vi "基于LabVIEW的光照度监测系统上位机软件设计.vi"() -> ()   [LabVIEW 2025]
uses:
  <vilib>/Instr/_visa.llb/VISA Configure Serial Port (Instr).vi
panel:
  out "转换为十进制数据":u32
  out "地址04的光亮度数据":dbl
  out "字符串显示·的十六进制数据":string
  out "无符号字节数组":u8[](array[numeric])
  out "十六进制整形字符串":string[](array[string])
  out "提取的从机地址04的亮度原始数据":string
  out "转换为十进制数据":u32
  out "地址03的光亮度数据":dbl
  out "字符串显示·的十六进制数据":string
  out "无符号字节数组":u8[](array[numeric])
  out "十六进制整形字符串":string[](array[string])
  out "提取的从机地址03的亮度原始数据":string
  out "转换为十进制数据":u32
  out "地址02的光亮度数据":dbl
  out "字符串显示的十六进制数据":string
  out "无符号字节数组":u8[](array[numeric])
  out "十六进制整形字符串":string[](array[string])
  out "提取的从机地址02的亮度原始数据":string
  out "转换为十进制数据":u32
  out "地址01的光亮度数据":dbl
  out "字符串显示的十六进制数据":string
  out "无符号字节数组":u8[](array[numeric])
  out "十六进制整形字符串":string[](array[string])
  out "提取的从机地址01的亮度原始数据":string
  out "地址03":u32(graph)
  out "地址04":u32(graph)
  in  "选择从机":u16(ring)=4 items=["从机04"=4, "从机03"=3, "从机02"=2, "从机01"=1]
  out "地址02":u32(graph)
  out "地址01":u32(graph)
  in  "停止采集":bool
  out "所有测量记录":string[][](table)
  in  "发送命令":string
  in  "波特率":u32=9600 caption="波特率(9600)"
  in  "选择串口":refnum<visa-resource-name>
  # "从机地址01："
  # "从机地址02："
  # "从机地址03："
  # "从机地址04："
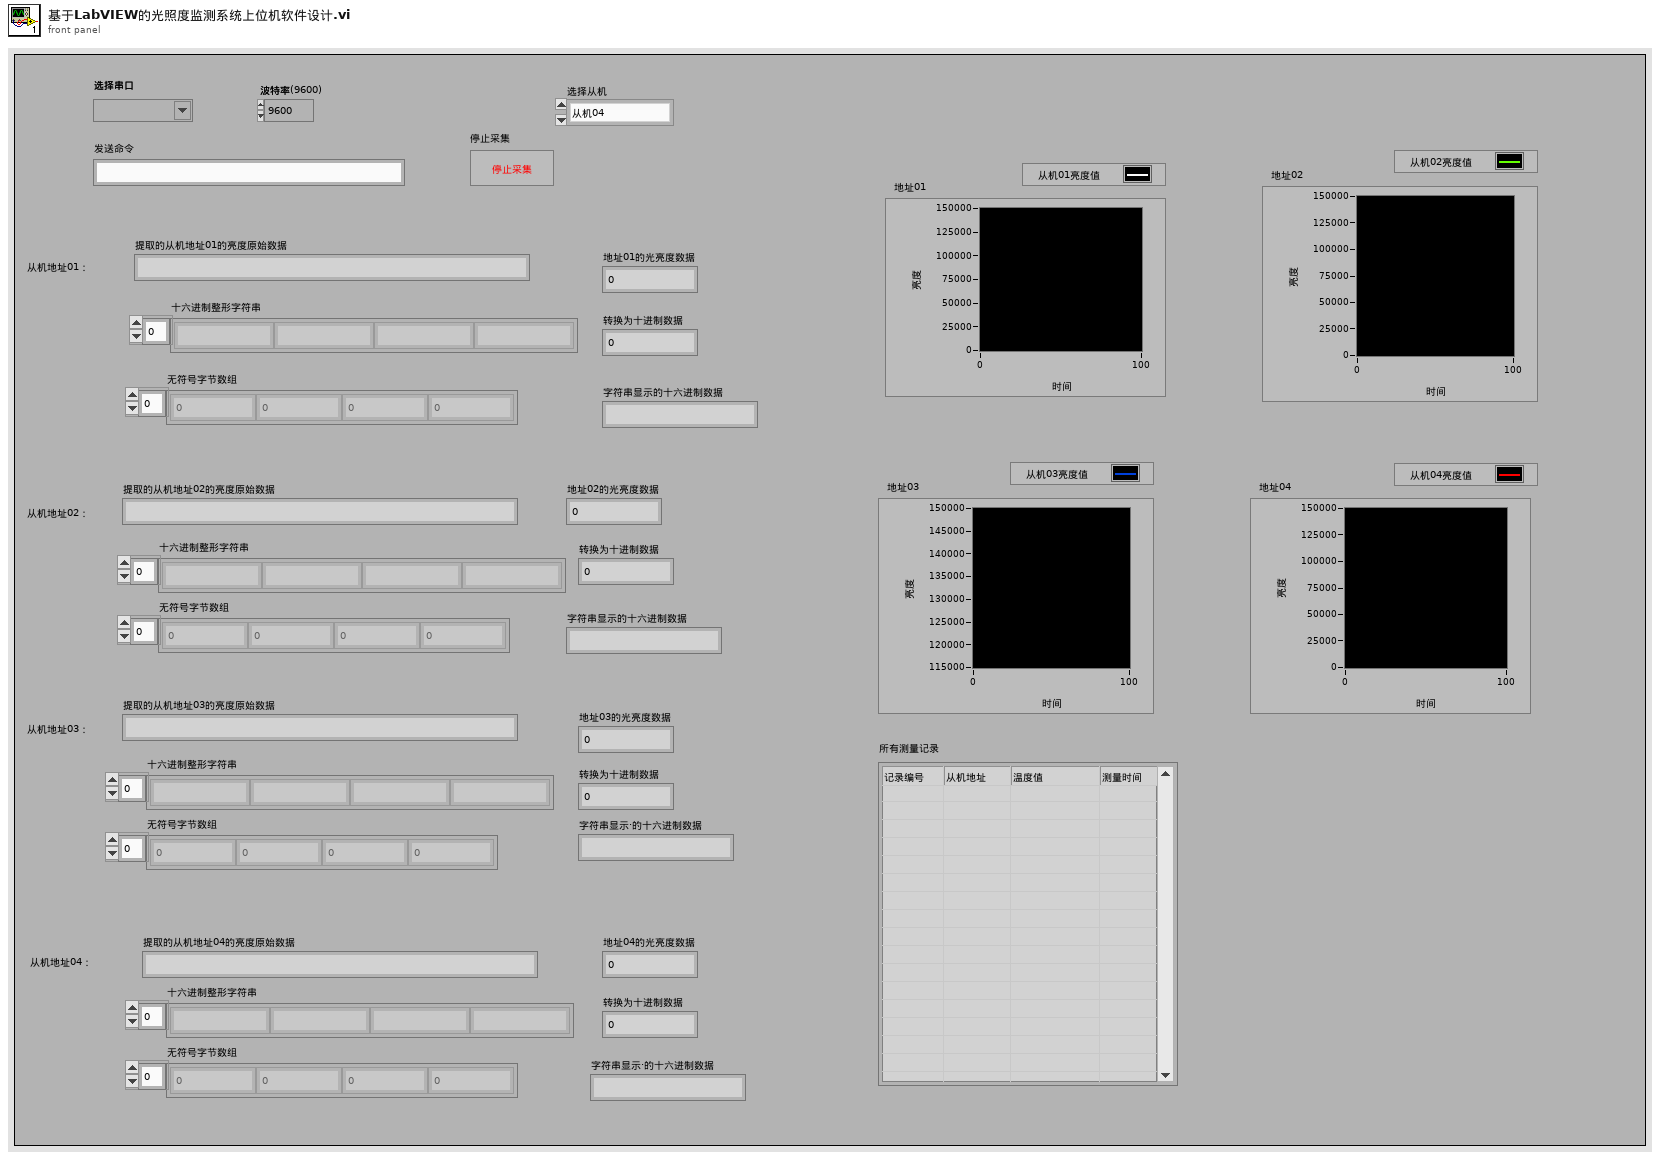
[diagram p1: front panel]
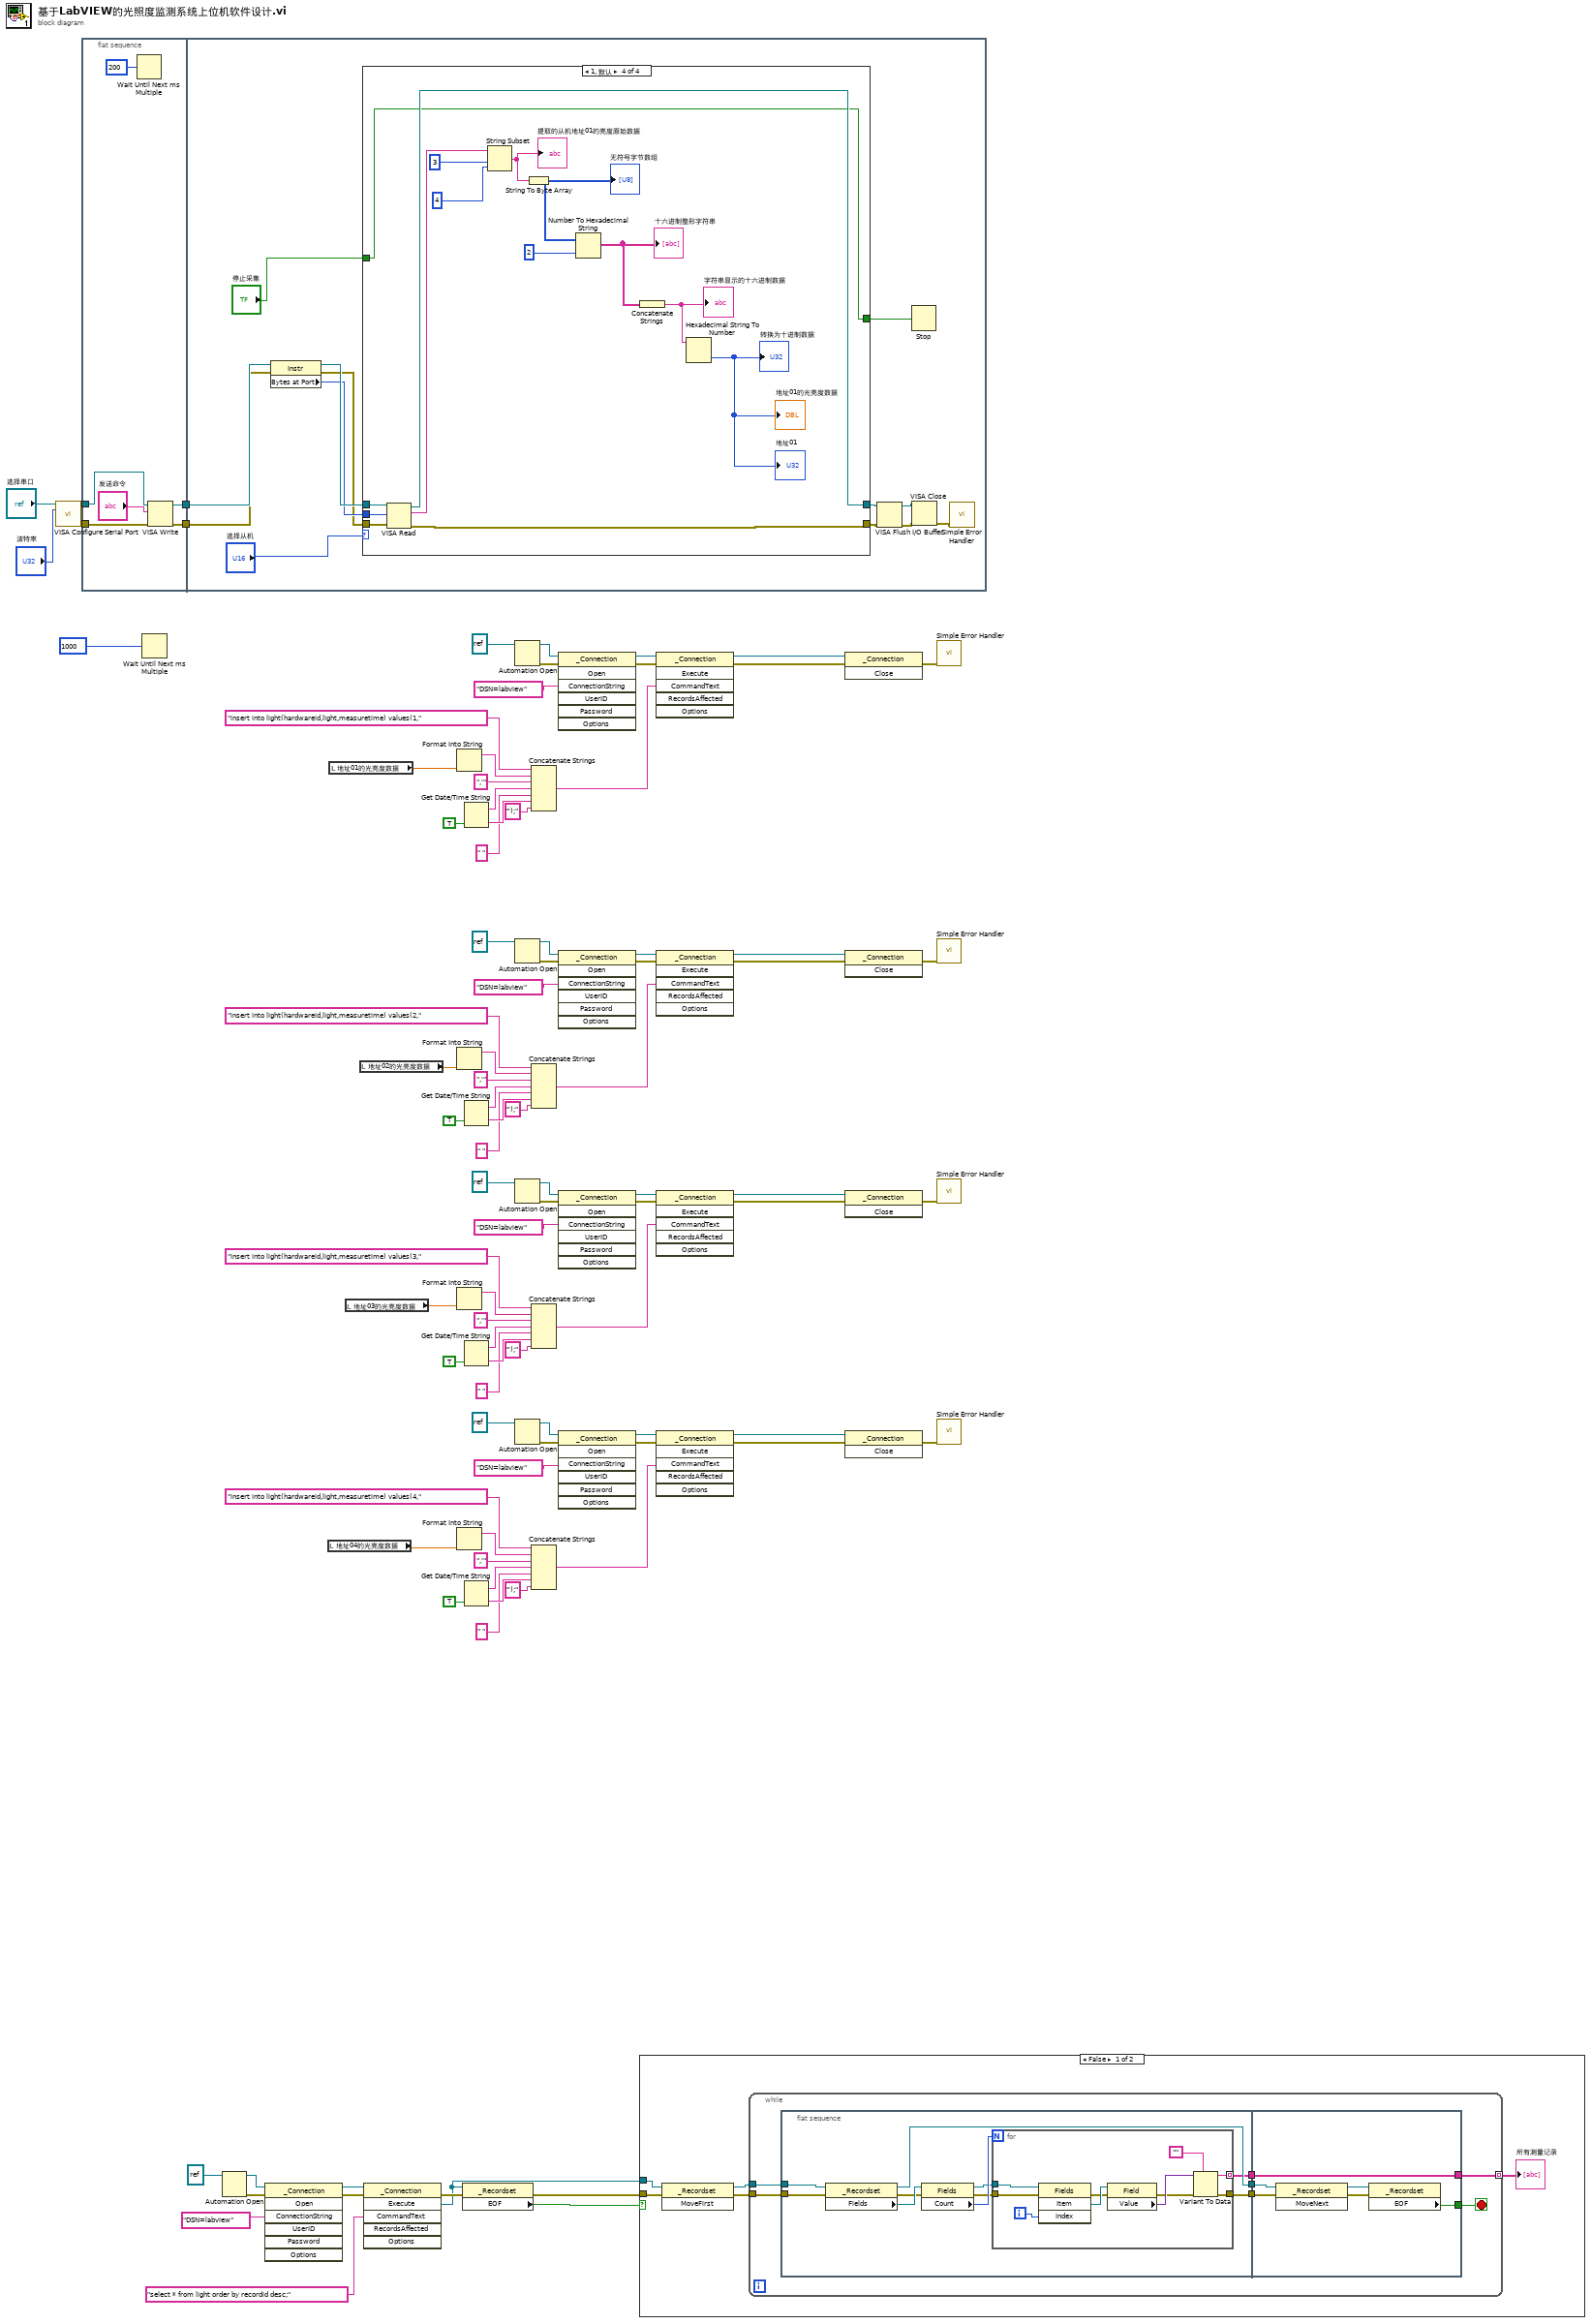
[diagram p0: block diagram]
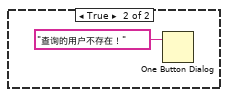
[diagram p2: hidden frame]
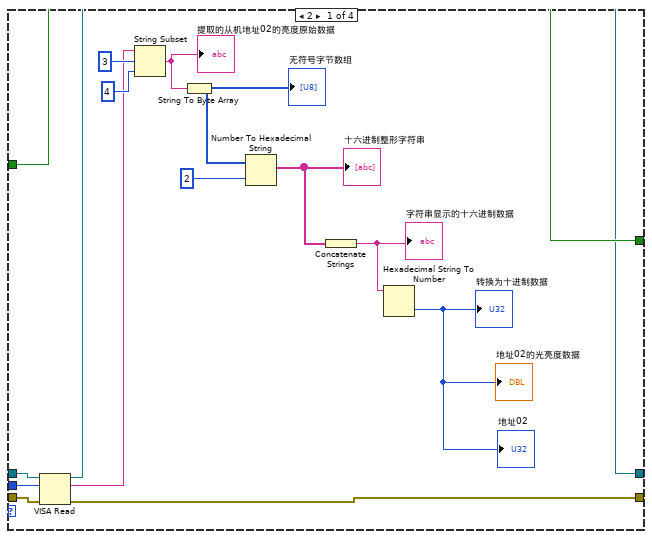
[diagram p3: hidden frame]
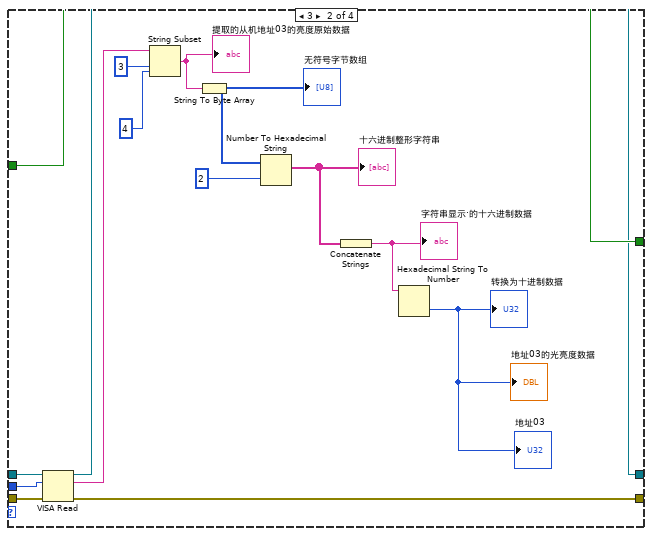
[diagram p4: hidden frame]
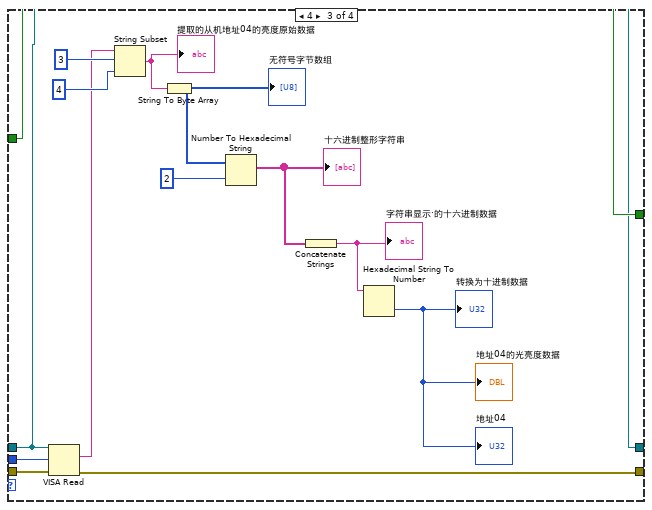
[diagram p5: hidden frame]
diagram:
  n1 = call-poly "VISA Configure Serial Port"("VISA resource name"="选择串口", "baud rate (9600)"="波特率") -> ("VISA resource name out"=w92:refnum<visa-resource-name>, "error out"=w91:errorcluster)  [unwired: 12 in]
  n2 = flat-sequence {
    tunnel: w92 -> [w99]
    tunnel: w91 -> [w98]
    tunnel: [w96] -> w90
    tunnel: [w95] -> w89
    tunnel: w90 -> [w113]
    tunnel: w89 -> [w112]
    frame #0 {
      n3 = Wait Until Next ms Multiple(millisecond multiple=u32 200 ("毫秒倍数")) -> ()  [unwired: 1 out]
      n4 = VISA Write(VISA resource name=w99, write buffer="发送命令", error in (no error)=w98) -> (VISA resource name out=w96:refnum<visa-resource-name>, error out=w95:errorcluster)  [unwired: 1 out]
    }
    frame #1 {
      n5 = property class="Instr"(reference=w113, error in=w112) -> (reference out=w111:refnum<visa-resource-name>, error out=w109:errorcluster, "Bytes at Port"=w110:u32)
      n6 = case shown="1, 默认" "选择从机" {
        tunnel: w111 -> [w128 w130 w145 w169]
        tunnel: w110 -> [w127 w135 w156 w168]
        tunnel: w109 -> [w126 w134 w155 w171]
        tunnel: [w116 w130 w145 w160] -> w105
        tunnel: [w125 w133 w154 w170] -> w104
        tunnel: [w124 w132 w146 w159] -> w101
        tunnel: "停止采集" -> [w124 w132 w146 w159]
        frame 2 {
          n7 = VISA Read(VISA resource name=w128, byte count=w127, error in (no error)=w126) -> (VISA resource name out=w116:refnum<visa-resource-name>, read buffer=w114:string, error out=w125:errorcluster)  [unwired: 1 out]
          n8 = String Subset(string=w114, offset (0)=3 ("偏移量(0)"), length (rest)=4 ("长度（剩余）")) -> (substring=w123:string)
          "提取的从机地址02的亮度原始数据" <- w123
          n9 = String To Byte Array(string=w123) -> (unsigned byte array=w122:u8[])
          "无符号字节数组" <- w122
          n10 = Number To Hexadecimal String(1:i16 2 ("宽度(-)"), 2:w122) -> (0:w121:string[])
          "十六进制整形字符串" <- w121
          n11 = Concatenate Strings(w121) -> (w120:string)
          "字符串显示的十六进制数据" <- w120
          n12 = Hexadecimal String To Number(string=w120) -> (number=→"地址02" →"地址02的光亮度数据" →"转换为十进制数据":u32)  [unwired: 2 in, 1 out]
        }
        frame 3 {
          n13 = VISA Read(VISA resource name=w130, byte count=w135, error in (no error)=w134) -> (read buffer=w129:string, error out=w133:errorcluster)  [unwired: 2 out]
          n14 = String Subset(string=w129, offset (0)=3 ("偏移量(0)"), length (rest)=4 ("长度（剩余）")) -> (substring=w142:string)
          "提取的从机地址03的亮度原始数据" <- w142
          n15 = String To Byte Array(string=w142) -> (unsigned byte array=w141:u8[])
          "无符号字节数组" <- w141
          n16 = Number To Hexadecimal String(1:i16 2 ("宽度(-)"), 2:w141) -> (0:w140:string[])
          "十六进制整形字符串" <- w140
          n17 = Concatenate Strings(w140) -> (w139:string)
          "字符串显示·的十六进制数据" <- w139
          n18 = Hexadecimal String To Number(string=w139) -> (number=→"地址03的光亮度数据" →"转换为十进制数据" →"地址03":u32)  [unwired: 2 in, 1 out]
        }
        frame 4 {
          n19 = VISA Read(VISA resource name=w145, byte count=w156, error in (no error)=w155) -> (read buffer=w143:string, error out=w154:errorcluster)  [unwired: 2 out]
          n20 = String Subset(string=w143, offset (0)=3 ("偏移量(0)"), length (rest)=4 ("长度（剩余）")) -> (substring=w153:string)
          "提取的从机地址04的亮度原始数据" <- w153
          n21 = String To Byte Array(string=w153) -> (unsigned byte array=w152:u8[])
          "无符号字节数组" <- w152
          n22 = Number To Hexadecimal String(1:i16 2 ("宽度(-)"), 2:w152) -> (0:w151:string[])
          "十六进制整形字符串" <- w151
          n23 = Concatenate Strings(w151) -> (w150:string)
          "字符串显示·的十六进制数据" <- w150
          n24 = Hexadecimal String To Number(string=w150) -> (number=→"地址04的光亮度数据" →"转换为十进制数据" →"地址04":u32)  [unwired: 2 in, 1 out]
        }
        frame 1, Default {
          n25 = VISA Read(VISA resource name=w169, byte count=w168, error in (no error)=w171) -> (VISA resource name out=w160:refnum<visa-resource-name>, read buffer=w157:string, error out=w170:errorcluster)  [unwired: 1 out]
          n26 = String Subset(string=w157, offset (0)=3 ("偏移量(0)"), length (rest)=4 ("长度（剩余）")) -> (substring=w164:string)
          "提取的从机地址01的亮度原始数据" <- w164
          n27 = String To Byte Array(string=w164) -> (unsigned byte array=w165:u8[])
          "无符号字节数组" <- w165
          n28 = Number To Hexadecimal String(1:i16 2 ("宽度(-)"), 2:w165) -> (0:w166:string[])
          "十六进制整形字符串" <- w166
          n29 = Concatenate Strings(w166) -> (w167:string)
          "字符串显示的十六进制数据" <- w167
          n30 = Hexadecimal String To Number(string=w167) -> (number=→"地址01" →"地址01的光亮度数据" →"转换为十进制数据":u32)  [unwired: 2 in, 1 out]
        }
      }
      n31 = VISA Flush I/O Buffer(VISA resource name=w105, error in (no error)=w104) -> (VISA resource name out=w106:refnum<visa-resource-name>, error out=w107:errorcluster)  [unwired: 1 in]
      n32 = Stop(stop? (T)=w101) -> ()
      n33 = VISA Close(VISA resource name=w106, error in (no error)=w107) -> (error out=w108:errorcluster)
      n34 = call <vilib>:"Simple Error Handler.vi"("error in (no error)"=w108) -> ()  [unwired: 4 in, 5 out]
    }
  }
  n35 = Wait Until Next ms Multiple(millisecond multiple=1000) -> ()  [unwired: 1 out]
  n36 = Automation Open(Automation Refnum=refnum<k7> refnum ("ADODB._Connection")) -> (Automation Refnum=w87:refnum<k7>, error out=w86:errorcluster)  [unwired: 3 in]
  n37 = invoke class="_Connection" method="Open"(reference=w87, error in=w86, "ConnectionString"="DSN=labview") -> (reference out=w84:refnum<k7>, error out=w83:errorcluster)  [unwired: 4 in, 5 out]
  n38 = local read "地址04的光亮度数据"() -> (w1:dbl)
  n39 = local read "地址01的光亮度数据"() -> (w4:dbl)
  n40 = local read "地址03的光亮度数据"() -> (w2:dbl)
  n41 = local read "地址02的光亮度数据"() -> (w3:dbl)
  n42 = invoke class="_Connection" method="Execute"(reference=w84, error in=w83, "CommandText"="select * from light order by recordid desc;") -> (error out=w81:errorcluster, "Execute"=w79:refnum<k7>)  [unwired: 3 in, 4 out]
  n43 = Format Into String(w4) -> (resulting string=w20:string)  [unwired: 3 in, 1 out]
  n44 = Format Into String(w3) -> (resulting string=w35:string)  [unwired: 3 in, 1 out]
  n45 = Format Into String(w2) -> (resulting string=w50:string)  [unwired: 3 in, 1 out]
  n46 = Format Into String(w1) -> (resulting string=w65:string)  [unwired: 3 in, 1 out]
  n47 = property class="_Recordset"(reference=w79, error in=w81) -> (error out=w78:errorcluster, "EOF"=w80:bool)  [unwired: 1 out]
  n48 = Get Date/Time String(want seconds? (F)=TRUE) -> (date string=w13:string, time string=w14:string)  [unwired: 2 in]
  n49 = Get Date/Time String(want seconds? (F)=TRUE) -> (date string=w28:string, time string=w29:string)  [unwired: 2 in]
  n50 = Get Date/Time String(want seconds? (F)=TRUE) -> (date string=w43:string, time string=w44:string)  [unwired: 2 in]
  n51 = Get Date/Time String(want seconds? (F)=TRUE) -> (date string=w58:string, time string=w59:string)  [unwired: 2 in]
  n52 = Automation Open(Automation Refnum=refnum<k7> refnum ("ADODB._Connection")) -> (Automation Refnum=w19:refnum<k7>, error out=w18:errorcluster)  [unwired: 3 in]
  n53 = Automation Open(Automation Refnum=refnum<k7> refnum ("ADODB._Connection")) -> (Automation Refnum=w34:refnum<k7>, error out=w33:errorcluster)  [unwired: 3 in]
  n54 = Automation Open(Automation Refnum=refnum<k7> refnum ("ADODB._Connection")) -> (Automation Refnum=w49:refnum<k7>, error out=w48:errorcluster)  [unwired: 3 in]
  n55 = Automation Open(Automation Refnum=refnum<k7> refnum ("ADODB._Connection")) -> (Automation Refnum=w64:refnum<k7>, error out=w63:errorcluster)  [unwired: 3 in]
  n56 = Concatenate Strings("insert into light(hardwareid,light,measuretime) values(1," ("CommandText"), w20, ",'" ("字符串"), w13, " " ("string"), w14, "');" ("string")) -> (w15:string)
  n57 = Concatenate Strings("insert into light(hardwareid,light,measuretime) values(2," ("CommandText"), w35, ",'" ("字符串"), w28, " " ("string"), w29, "');" ("string")) -> (w30:string)
  n58 = Concatenate Strings("insert into light(hardwareid,light,measuretime) values(3," ("CommandText"), w50, ",'" ("字符串"), w43, " " ("string"), w44, "');" ("string")) -> (w45:string)
  n59 = Concatenate Strings("insert into light(hardwareid,light,measuretime) values(4," ("CommandText"), w65, ",'" ("字符串"), w58, " " ("string"), w59, "');" ("string")) -> (w60:string)
  n60 = invoke class="_Connection" method="Open"(reference=w19, error in=w18, "ConnectionString"="DSN=labview") -> (reference out=w17:refnum<k7>, error out=w16:errorcluster)  [unwired: 4 in, 5 out]
  n61 = invoke class="_Connection" method="Open"(reference=w34, error in=w33, "ConnectionString"="DSN=labview") -> (reference out=w32:refnum<k7>, error out=w31:errorcluster)  [unwired: 4 in, 5 out]
  n62 = invoke class="_Connection" method="Open"(reference=w49, error in=w48, "ConnectionString"="DSN=labview") -> (reference out=w47:refnum<k7>, error out=w46:errorcluster)  [unwired: 4 in, 5 out]
  n63 = invoke class="_Connection" method="Open"(reference=w64, error in=w63, "ConnectionString"="DSN=labview") -> (reference out=w62:refnum<k7>, error out=w61:errorcluster)  [unwired: 4 in, 5 out]
  n64 = case shown="False" w80 {
    tunnel: w79 -> [w176 _]
    tunnel: w78 -> [w175 _]
    frame False {
      n65 = invoke class="_Recordset" method="MoveFirst"(reference=w176, error in=w175) -> (reference out=w173:refnum<k7>, error out=w174:errorcluster)  [unwired: 1 in, 1 out]
      n66 = while {
        tunnel: w174 -> [w181]
        tunnel: w173 -> [w180]
        tunnel: [w177] -> w172 mode=indexing
        stop <- w179 stop-if-true
        n67 = flat-sequence {
          tunnel: w180 -> [w193]
          tunnel: w181 -> [w192]
          tunnel: [w186] -> w183
          tunnel: [w185] -> w182
          tunnel: [w184] -> w178
          tunnel: w183 -> [w207]
          tunnel: w182 -> [w206]
          tunnel: [w205] -> w179
          tunnel: w178 -> [w204]
          tunnel: [w204] -> w177
          frame #0 {
            n68 = property class="_Recordset"(reference=w193, error in=w192) -> (reference out=w185:refnum<k7>, error out=w190:errorcluster, "Fields"=w191:refnum<k7>)
            n69 = property class="Fields"(reference=w191, error in=w190) -> (reference out=w188:refnum<k7>, error out=w187:errorcluster, "Count"=w189:i32)
            n70 = for {
              N: w189 -> [_]
              tunnel: w188 -> [w198]
              tunnel: w187 -> [w197]
              tunnel: [w195] -> w184 mode=indexing
              tunnel: [w194] -> w186
              i -> [w196]
              n71 = invoke class="Fields" method="Item"(reference=w198, error in=w197, "Index"=w196) -> (error out=w202:errorcluster, "Item"=w203:refnum<k7>)  [unwired: 1 in, 2 out]
              n72 = property class="Field"(reference=w203, error in=w202) -> (error out=w199:errorcluster, "Value"=w200:variant)  [unwired: 1 out]
              n73 = Variant To Data(error in=w199, type="", Variant=w200) -> (data=w195:string, error out=w194:errorcluster)
            }
          }
          frame #1 {
            n74 = invoke class="_Recordset" method="MoveNext"(reference=w206, error in=w207) -> (reference out=w209:refnum<k7>, error out=w208:errorcluster)  [unwired: 1 in, 1 out]
            n75 = property class="_Recordset"(reference=w209, error in=w208) -> ("EOF"=w205:bool)  [unwired: 2 out]
          }
        }
      }
      "所有测量记录" <- w172
    }
    frame True {
      n76 = One Button Dialog(message="查询的用户不存在！") -> ()  [unwired: 1 in, 1 out]
    }
  }
  n77 = invoke class="_Connection" method="Execute"(reference=w17, error in=w16, "CommandText"=w15) -> (reference out=w67:refnum<k7>, error out=w66:errorcluster)  [unwired: 3 in, 4 out]
  n78 = invoke class="_Connection" method="Execute"(reference=w32, error in=w31, "CommandText"=w30) -> (reference out=w70:refnum<k7>, error out=w69:errorcluster)  [unwired: 3 in, 4 out]
  n79 = invoke class="_Connection" method="Execute"(reference=w47, error in=w46, "CommandText"=w45) -> (reference out=w73:refnum<k7>, error out=w72:errorcluster)  [unwired: 3 in, 4 out]
  n80 = invoke class="_Connection" method="Execute"(reference=w62, error in=w61, "CommandText"=w60) -> (reference out=w76:refnum<k7>, error out=w75:errorcluster)  [unwired: 3 in, 4 out]
  n81 = invoke class="_Connection" method="Close"(reference=w67, error in=w66) -> (error out=w68:errorcluster)  [unwired: 1 in, 2 out]
  n82 = invoke class="_Connection" method="Close"(reference=w70, error in=w69) -> (error out=w71:errorcluster)  [unwired: 1 in, 2 out]
  n83 = invoke class="_Connection" method="Close"(reference=w73, error in=w72) -> (error out=w74:errorcluster)  [unwired: 1 in, 2 out]
  n84 = invoke class="_Connection" method="Close"(reference=w76, error in=w75) -> (error out=w77:errorcluster)  [unwired: 1 in, 2 out]
  n85 = call <vilib>:"Simple Error Handler.vi"("error in (no error)"=w68) -> ()  [unwired: 4 in, 5 out]
  n86 = call <vilib>:"Simple Error Handler.vi"("error in (no error)"=w71) -> ()  [unwired: 4 in, 5 out]
  n87 = call <vilib>:"Simple Error Handler.vi"("error in (no error)"=w74) -> ()  [unwired: 4 in, 5 out]
  n88 = call <vilib>:"Simple Error Handler.vi"("error in (no error)"=w77) -> ()  [unwired: 4 in, 5 out]
